vi "Test_Observe_NoPublication_Timeout.vi"(8 "error in (no error)":errorcluster, 11 "TestObservation In":refnum<class "TestPubSubRouting.lvclass">) -> (0 "error out":errorcluster, 3 "TestObservation Out":refnum<class "TestPubSubRouting.lvclass">)   [LabVIEW 2017, in "TestPubSubRouting.lvlib" / "TestPubSubRouting.lvclass"]
uses:
  TestPubSubRouting.lvclass
  Source/Framework/Mediator/Mediator/Mediator.lvclass
  C:/Git/mva-framework/Source/Framework/IMediator/IMediator/IMediator.lvclass
  Source/Framework/IObserver/IObserver/IObserver.lvclass/IObserver.ctl
  Source/Framework/IMediator/IMediator/IMediator.lvclass/IMediator.ctl
  Source/Framework/IViewModel/IViewModel/IViewModel.lvclass/IViewModel.ctl
  Source/Framework/IViewManager/IViewManager Messages/Launch Nested Views Msg/Launch Nested Views Msg.lvclass/Launch Nested Views Msg.ctl
  Source/Framework/IViewManager/IViewManager/IViewManager.lvclass/IViewManager.ctl
  <vilib>/ActorFramework/Message Enqueuer/Message Enqueuer.lvclass/Message Enqueuer.ctl
  41be6b66-6851-409e-b7f3-4ca1eaa927d9.vi
  Source/Framework/IObserver/IObserver/Configure Observer Logging.vi
  Source/Framework/IViewModel/IViewModel/Write Startup Model-View Configuration.vi
  Source/Framework/IMediator/IMediator/Configure Mediator.vi
  <vilib>/ActorFramework/Message Enqueuer/Enqueue.vi
  Source/Framework/IViewManager/IViewManager Messages/Launch Nested Views Msg/Pack Launch Nested Views Msg.vi
  Source/Framework/IViewManager/IViewManager/Write Startup Launch Nested Views Msg.vi
  ObservingModel/ObservingModel.lvclass
  C:/Git/mva-framework/Source/Framework/IObserver/IObserver/IObserver.lvclass
  C:/Git/mva-framework/Source/Framework/IModel/IModel/IModel.lvclass
  ObservingViewable/ObservingViewable.lvclass
  C:/Git/mva-framework/Source/Framework/IViewable/IViewable/IViewable.lvclass
  ObservingViewModel/ObservingViewModel.lvclass
  C:/Git/mva-framework/Source/Framework/IViewModel/IViewModel/IViewModel.lvclass
  C:/Program Files (x86)/National Instruments/LabVIEW 2017/vi.lib/ActorFramework/Actor/Actor.lvclass
  Source/Framework/IViewModel/IViewModel/IViewModel.lvclass
  C:/Git/mva-framework/Source/Framework/IViewManager/IViewManager/IViewManager.lvclass
  <vilib>/ActorFramework/Stop Msg/Stop Msg.lvclass
  C:/Program Files (x86)/National Instruments/LabVIEW 2017/vi.lib/ActorFramework/Message/Message.lvclass
  <vilib>/ActorFramework/Message Priority Queue/Priority Enqueue.vi
  gpm_packages/@cs/event-logger/Source/Composed Log/LoggerReference/LoggerReference.lvclass
  Source/Framework/IMediator/IMediatorBusMonitor/MediatorBusMonitor/IMediatorBusMonitor.lvclass
  gpm_packages/@cs/event-logger/Source/Text File Sink/Text File Sink.lvclass
  Source/Framework/IViewable/IApplicationStyle/IApplicationStyle.lvclass
  Source/Framework/IViewManager/IViewManager Messages/Launch Nested Views Msg/Launch Nested Views Msg.lvclass
  <vilib>/ActorFramework/Actor/Actor.lvclass
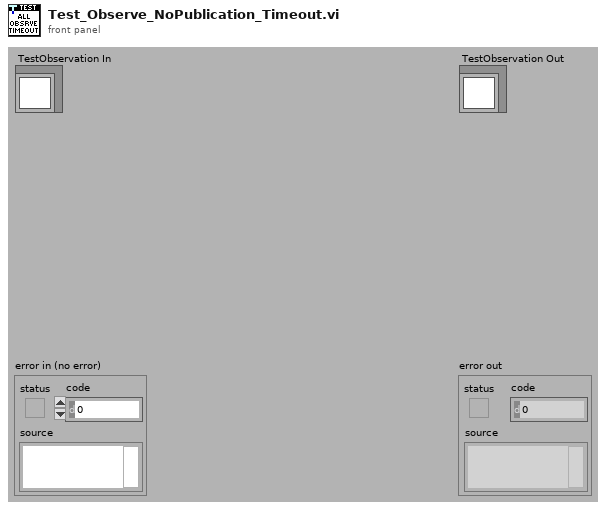
[diagram p1: front panel]
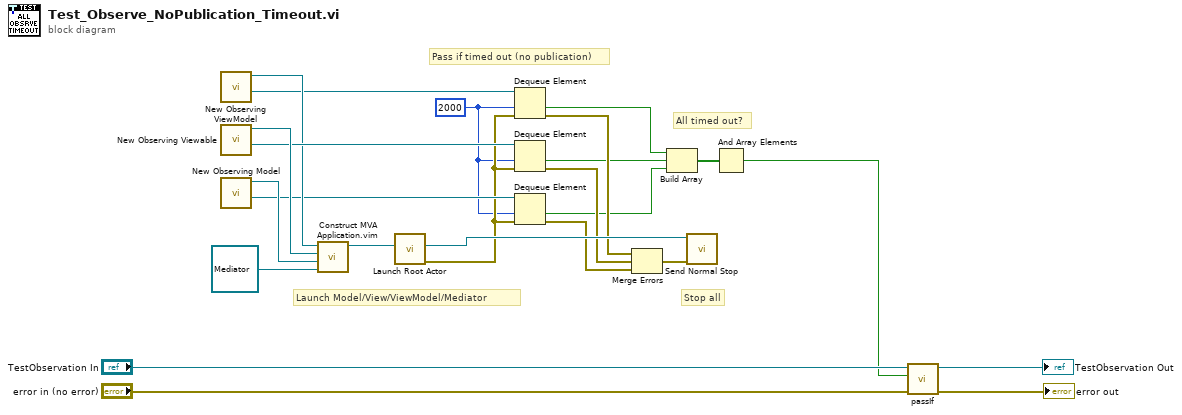
[diagram p0: block diagram]
diagram:
  w10 = 2000 ("timeout in ms (-1)")
  # "All timed out?"
  # "Stop all"
  # "Launch Model/View/ViewModel/Mediator"
  # "Pass if timed out (no publication)"
  n1 = call "New Observing ViewModel.vi"() -> ("Test Reply Queue"=w13:refnum<queue>, "ObservingViewModel Out"=w15:refnum<class "ObservingViewModel.lvclass">)  [unwired: 10 in]
  n2 = call "New Observing Viewable.vi"() -> ("Test Reply Queue"=w17:refnum<queue>, "ObservingViewable out"=w18:refnum<class "ObservingViewable.lvclass">)  [unwired: 10 in]
  n3 = call "New Observing Model.vi"() -> ("Test Reply Queue"=w12:refnum<queue>, "ObservingModel Out"=w14:refnum<class "ObservingModel.lvclass">)  [unwired: 10 in]
  n4 = call "Construct MVA Application.vim"("Mediator Type"=refnum<class "Mediator.lvclass"> refnum ("Mediator.lvlib:Mediator.lvclass"), "Model Type"=w14, "Startup View Configuration"=w18, "IViewModel In"=w15) -> ("IViewModel Out"=w19:refnum<class "ObservingViewModel.lvclass">)  [unwired: 7 in]
  n5 = call <vilib>:"Launch Root Actor.vi"("Actor"=w19) -> ("error out"=w11:errorcluster, "Actor's Enqueuer"=w16:refnum<class "Message Enqueuer.lvclass">)  [unwired: 9 in]
  n6 = Dequeue Element(queue=w13, timeout in ms (-1)=w10, error in (no error)=w11) -> (timed out?=w4:bool, error out=w9:errorcluster)  [unwired: 2 out]
  n7 = Dequeue Element(queue=w17, timeout in ms (-1)=w10, error in (no error)=w11) -> (timed out?=w3:bool, error out=w8:errorcluster)  [unwired: 2 out]
  n8 = Dequeue Element(queue=w12, timeout in ms (-1)=w10, error in (no error)=w11) -> (timed out?=w2:bool, error out=w7:errorcluster)  [unwired: 2 out]
  n9 = Merge Errors(w9, w8, w7) -> (w6:errorcluster)
  n10 = Build Array(w4, w3, w2) -> (w5:bool[])
  n11 = call <vilib>:"Send Normal Stop.vi"("error in (no error)"=w6, "Message Enqueuer"=w16) -> ()  [unwired: 9 in, 1 out]
  n12 = And Array Elements(Boolean array=w5) -> (logical AND=w1:bool)
  n13 = call-dynamic "passIf.vi"("error in (no error)"="error in (no error)", "pass"=w1, "TestCase in"="TestObservation In") -> ("error out"=→"error out":errorcluster, "TestCase out"=→"TestObservation Out":refnum<class "TestPubSubRouting.lvclass">)  [unwired: 7 in]
